vi "Begin.vi"() -> (0 "error out":errorcluster, 1 "CameraDevRef":T1)   [LabVIEW 2011]
doc: "Called before other user functions, this VI is expected to open initial I/O refnums, load in file data, and do all program initialization. Notice that the <B>error out</B> terminal is simply used for data flow. Wiring it to other structures or subVIs ensures that this VI runs first."
uses:
  <vilib>/Rock Robotics/WPI/Camera/WPI_CameraDevRef.ctl
  <vilib>/Rock Robotics/SystemInterfaces/DIO/FPGA_DIOPWMChannel.ctl
  <vilib>/Rock Robotics/WPI/Joystick/WPI_JoystickDeviceEnum.ctl
  <vilib>/Rock Robotics/SystemInterfaces/Typedef/FPGA_TypedefDigitalModule.ctl
  <vilib>/Rock Robotics/SystemInterfaces/DIO/FPGA_DIORelayChannel.ctl
  <vilib>/Rock Robotics/WPI/MotorControl/WPI_MotorControlOpen Victor.vi
  <vilib>/Rock Robotics/WPI/MotorControl/WPI_MotorControlOpen Jaguar.vi
  Robot Global Data.vi
panel:
  out "Global: Auton Files":string[](array[string])
  out "Global: Auton Array":dbl[][](array[numeric])
  out "Global: Current Auton File":string
  out "Global: Number of Auton Files":i64
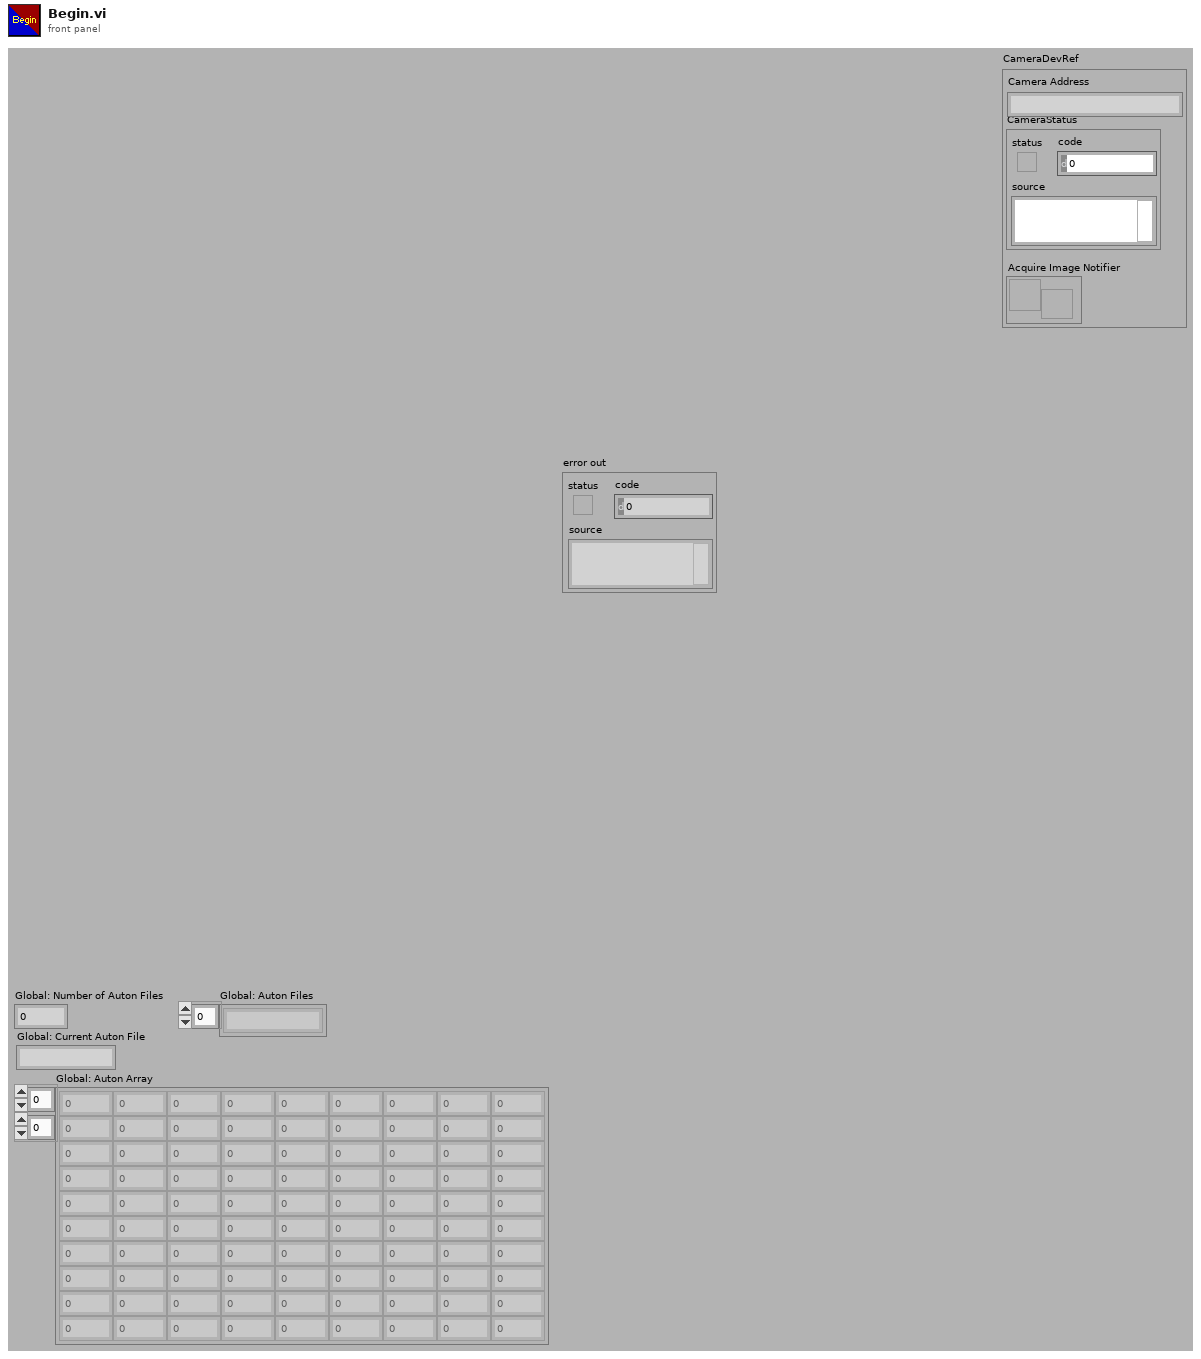
[diagram p1: front panel]
types:
  T1 = typedef "WPI_CameraDevRef.ctl" = cluster{"Camera Address":string, "CameraStatus":errorcluster, "Acquire Image Notifier":refnum<notifier>}
  T2 = typedef "FPGA_DIORelayChannel.ctl" = enum8{"Relay 1", "Relay 2", "Relay 3", "Relay 4", "Relay 5", "Relay 6", "Relay 7", "Relay 8", "Invalid"}
  T3 = typedef "FPGA_TypedefDigitalModule.ctl" = enum16{"Digital Module 1", "Digital Module 2"}
  T4 = typedef "WPI_JoystickDeviceEnum.ctl" = enum16{"USB 1", "USB 2", "USB 3", "USB 4", "Kinect 1", "Kinect 2"}
  T5 = typedef "FPGA_DIOPWMChannel.ctl" = enum8{"PWM 1", "PWM 2", "PWM 3", "PWM 4", "PWM 5", "PWM 6", "PWM 7", "PWM 8", "PWM 9", "PWM 10", "Invalid"}
  T6 = typedef "WPI_CameraImageSize.ctl" = enum16{"640x480", "320x240", "160x120"}
  T7 = cluster{"fps":i32, "compression":i32, "Image Size":T6}
  T8 = typedef "WPI_CameraWhite Balance Values.ctl" = enum16{"Auto", "Fixed indoor", "Fixed outdoor 1", "Fixed outdoor 2", "Fixed fluorescent 1", "Fixed fluorescent 2", "Hold current"}
  T9 = typedef "WPI_ServoDeviceRef.ctl" = cluster{"DeviceStatus":errorcluster, "Digital Module":T3, "PWM Channel":T5, "DeadBand":T10}
  T10 = typedef "WPI_PWMDeadband.ctl" = cluster{"Name":string, "maxPositivePwm":i32, "minPositivePwm":i32, "centerPwm":i32, "maxNegativePwm":i32, "minNegativePwm":i32, "angularRange":u16}
  T11 = typedef "WPI_MotorControlDeviceRef.ctl" = cluster{"DeviceStatus":errorcluster, "Type":enum16{"PWM", "CAN"}, "PWM":cluster{"Digital Module":T3, "PWM Channel":T5, "DeadBand":T10}, "CAN":cluster{"Device Number":u8, "Control Mode":T12, "Semaphore":T13, "Max Vout":dbl}, "Invert":bool, "TransformRef":T14, "InvTransformRef":T14}
  T12 = typedef "WPI_CANJaguar_ControlMode.ctl" = enum8{"Percent VBus", "Current", "Speed", "Position", "Voltage"}
  T13 = typedef "Semaphore RefNum" = refnum<k1>
  T14 = typedef "WPI_PWMTransform_ConPane.ctl" = refnum<vi>
  T15 = typedef "WPI_CameraExposure Values.ctl" = enum16{"Auto", "Flicker-free 50 Hz", "Flicker-free 60 Hz", "Hold current"}
  T16 = typedef "WPI_RelayDevRef.ctl" = cluster{"DevStatus":errorcluster, "Relay Channel":T2, "Digital Module":T3, "Relay Direction":T17}
  T17 = typedef "WPI_RelayDirection.ctl" = enum16{"Both directions", "Forward only", "Reverse only"}
  T18 = typedef "WPI_JoystickDevRef.ctl" = cluster{"Device":T4}
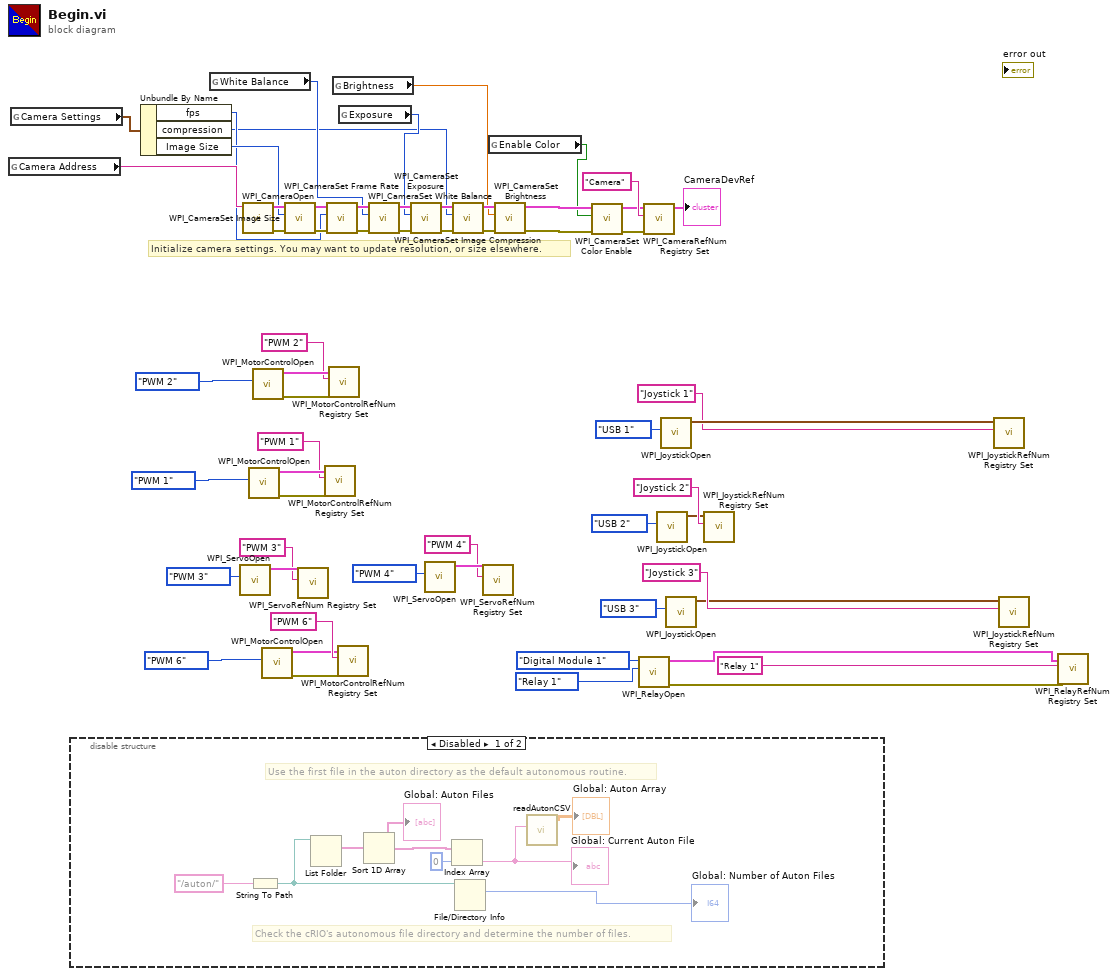
[diagram p0: block diagram]
diagram:
  # "Initialize camera settings. You may want to update resolution, or size elsewhere."
  n1 = global read "Robot Global Data.vi" "Camera Address"() -> (w46:string)
  n2 = global read "Robot Global Data.vi" "Camera Settings"() -> (w13:T7)
  n3 = disable-structure shown="Disabled" {
    frame Disabled {
      # "Check the cRIO's autonomous file directory and determine the number of files."
      # "Use the first file in the auton directory as the default autonomous routine."
      n4 = String To Path(string="/auton/") -> (path=w66:path)
      n5 = List Folder(path=w66) -> (filenames=w65:string[])  [unwired: 1 in, 5 out]
      n6 = Sort 1D Array(array=w65) -> (sorted array=w63:string[])
      "Global: Auton Files" <- w63
      n7 = Index Array(array=w63, index=0) -> (element=w61:string)
      "Global: Current Auton File" <- w61
      n8 = File/Directory Info(path=w66) -> (size=→"Global: Number of Auton Files":i64)  [unwired: 1 in, 6 out]
      n9 = call "readAutonCSV.vi"("AutonFile"=w61) -> ("AutonArray"=→"Global: Auton Array":dbl[][])  [unwired: 7 in]
    }
    frame Enabled {
    }
  }
  n10 = Unbundle By Name(w13) -> ("fps"=w11:i32, "compression"=w8:i32, "Image Size"=w12:T6)
  n11 = global read "Robot Global Data.vi" "White Balance"() -> (w10:T8)
  n12 = call <vilib>:"WPI_ServoOpen.vi"("PWM Channel"=FPGA_DIOPWMChannel."PWM 3") -> ("ServoDeviceRef"=w32:T9)  [unwired: 9 in, 1 out]
  n13 = call <vilib>:"WPI_CameraOpen.vi"("Camera Address"=w46) -> ("error out"=w52:errorcluster, "CameraDevRef"=w53:T1)  [unwired: 1 in, 8 out]
  n14 = call-poly <vilib>:"WPI_MotorControlOpen.vi"("PWM Channel"=FPGA_DIOPWMChannel."PWM 1") -> ("error out"=w38:errorcluster, "MotorControlDeviceRef"=w41:T11)  [unwired: 9 in]
  n15 = call-poly <vilib>:"WPI_MotorControlOpen.vi"("PWM Channel"=FPGA_DIOPWMChannel."PWM 2") -> ("error out"=w39:errorcluster, "MotorControlDeviceRef"=w44:T11)  [unwired: 9 in]
  n16 = call-poly <vilib>:"WPI_MotorControlOpen.vi"("PWM Channel"=FPGA_DIOPWMChannel."PWM 6") -> ("error out"=w27:errorcluster, "MotorControlDeviceRef"=w25:T11)  [unwired: 9 in]
  n17 = call <vilib>:"WPI_CameraSet Image Size.vi"("error in (no error)"=w52, "Image Size"=w12, "CameraDevRef"=w53) -> ("error out"=w51:errorcluster, "CameraDevRef Out"=w54:T1)  [unwired: 7 out]
  n18 = call <vilib>:"WPI_ServoRefNum Registry Set.vi"("refnum name"="PWM 3", "ServoDeviceRef"=w32) -> ()  [unwired: 8 in, 2 out]
  n19 = call <vilib>:"WPI_MotorControlRefNum Registry Set.vi"("error in (no error)"=w38, "refnum name"="PWM 1", "MotorControlDevRef"=w41) -> ()  [unwired: 7 in, 2 out]
  n20 = call <vilib>:"WPI_CameraSet Frame Rate.vi"("error in (no error)"=w51, "Frame Rate (fps)"=w11, "CameraDevRef"=w54) -> ("error out"=w50:errorcluster, "CameraDevRef Out"=w56:T1)  [unwired: 7 out]
  n21 = call <vilib>:"WPI_MotorControlRefNum Registry Set.vi"("error in (no error)"=w39, "refnum name"="PWM 2", "MotorControlDevRef"=w44) -> ()  [unwired: 7 in, 2 out]
  n22 = global read "Robot Global Data.vi" "Brightness"() -> (w7:dbl)
  n23 = call <vilib>:"WPI_MotorControlRefNum Registry Set.vi"("error in (no error)"=w27, "refnum name"="PWM 6", "MotorControlDevRef"=w25) -> ()  [unwired: 7 in, 2 out]
  n24 = global read "Robot Global Data.vi" "Exposure"() -> (w9:T15)
  n25 = call <vilib>:"WPI_CameraSet White Balance.vi"("error in (no error)"=w50, "White Balance"=w10, "CameraDevRef"=w56) -> ("error out"=w49:errorcluster, "CameraDevRef Out"=w55:T1)  [unwired: 7 out]
  n26 = call <vilib>:"WPI_CameraSet Exposure.vi"("error in (no error)"=w49, "Exposure"=w9, "CameraDevRef"=w55) -> ("error out"=w48:errorcluster, "CameraDevRef Out"=w58:T1)  [unwired: 7 out]
  n27 = call <vilib>:"WPI_ServoOpen.vi"("PWM Channel"=FPGA_DIOPWMChannel."PWM 4") -> ("ServoDeviceRef"=w30:T9)  [unwired: 9 in, 1 out]
  n28 = call <vilib>:"WPI_CameraSet Image Compression.vi"("error in (no error)"=w48, "Compression"=w8, "CameraDevRef"=w58) -> ("error out"=w47:errorcluster, "CameraDevRef Out"=w57:T1)  [unwired: 7 out]
  n29 = call <vilib>:"WPI_ServoRefNum Registry Set.vi"("refnum name"="PWM 4", "ServoDeviceRef"=w30) -> ()  [unwired: 8 in, 2 out]
  n30 = global read "Robot Global Data.vi" "Enable Color"() -> (w2:bool)
  n31 = call <vilib>:"WPI_CameraSet Brightness.vi"("error in (no error)"=w47, "Brightness"=w7, "CameraDevRef"=w57) -> ("error out"=w5:errorcluster, "CameraDevRef Out"=w6:T1)  [unwired: 7 out]
  n32 = call <vilib>:"WPI_CameraSet Color Enable.vi"("error in (no error)"=w5, "Color Enabled"=w2, "CameraDevRef"=w6) -> ("error out"=w3:errorcluster, "CameraDevRef Out"=w4:T1)  [unwired: 7 in]
  n33 = call <vilib>:"WPI_RelayOpen.vi"("Relay Channel"=FPGA_DIORelayChannel."Relay 1", "Digital Module (Module 1)"=FPGA_TypedefDigitalModule."Digital Module 1") -> ("error out"=w16:errorcluster, "RelayDevRef"=w17:T16)  [unwired: 8 in]
  n34 = call <vilib>:"WPI_CameraRefNum Registry Set.vi"("error in (no error)"=w3, "refnum name"="Camera", "CameraDevRef"=w4) -> ("CameraDevRef"=→"CameraDevRef":T1)  [unwired: 8 out]
  n35 = call <vilib>:"WPI_JoystickOpen.vi"("JoystickDevice"=WPI_JoystickDeviceEnum."USB 2") -> ("JoystickDevRef"=w34:T18)  [unwired: 10 in]
  n36 = call <vilib>:"WPI_JoystickOpen.vi"("JoystickDevice"=WPI_JoystickDeviceEnum."USB 1") -> ("JoystickDevRef"=w37:T18)  [unwired: 10 in]
  n37 = call <vilib>:"WPI_JoystickOpen.vi"("JoystickDevice"=WPI_JoystickDeviceEnum."USB 3") -> ("JoystickDevRef"=w22:T18)  [unwired: 10 in]
  n38 = call <vilib>:"WPI_JoystickRefNum Registry Set.vi"("refnum name"="Joystick 2", "JoystickDevRef"=w34) -> ()  [unwired: 8 in, 2 out]
  n39 = call <vilib>:"WPI_JoystickRefNum Registry Set.vi"("refnum name"="Joystick 1", "JoystickDevRef"=w37) -> ()  [unwired: 8 in, 2 out]
  n40 = call <vilib>:"WPI_JoystickRefNum Registry Set.vi"("refnum name"="Joystick 3", "JoystickDevRef"=w22) -> ()  [unwired: 8 in, 2 out]
  n41 = call <vilib>:"WPI_RelayRefNum Registry Set.vi"("error in (no error)"=w16, "refnum name"="Relay 1", "RelayDevRef"=w17) -> ()  [unwired: 7 in, 2 out]
